vi "Waveform Cluster to Array.vi"(10 "Waveform Cluster":T1) -> (1 "Lengths":i32[](array[numeric]), 2 "Concatenated Waveforms":waveform(dbl)[](array[waveform]))   [LabVIEW 2019, in "Instrument.Lockin.lvlib" / "Instrument.DAQ.lvclass"]
uses:
  Instrument.DAQ.lvclass
  Typedefs/PublicEvents--DAQ.getWaveforms.ctl
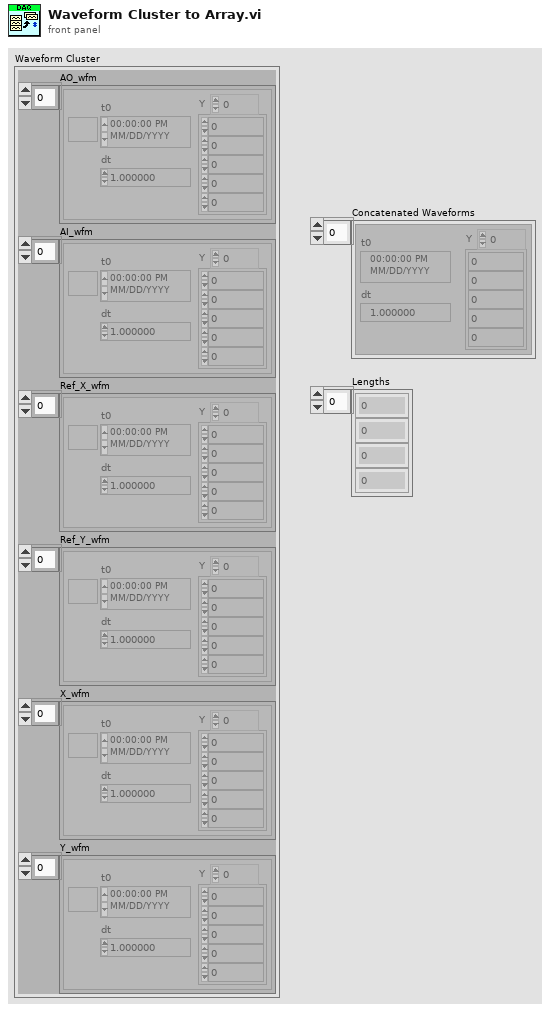
[diagram p1: front panel]
types:
  T1 = typedef "Instrument.Lockin.lvlib/Instrument.DAQ.lvclass/PublicEvents--DAQ.getWaveforms.ctl" = cluster{"AO_wfm":waveform(dbl)[], "AI_wfm":waveform(dbl)[], "Ref_X_wfm":waveform(dbl)[], "Ref_Y_wfm":waveform(dbl)[], "X_wfm":waveform(dbl)[], "Y_wfm":waveform(dbl)[]}
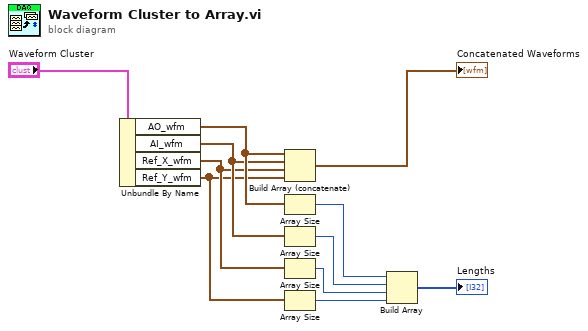
[diagram p0: block diagram]
diagram:
  n1 = Unbundle By Name("Waveform Cluster") -> ("AO_wfm"=w4:waveform(dbl)[], "AI_wfm"=w3:waveform(dbl)[], "Ref_X_wfm"=w2:waveform(dbl)[], "Ref_Y_wfm"=w1:waveform(dbl)[])
  n2 = Build Array (concatenate)(w4, w3, w2, w1) -> (→"Concatenated Waveforms":waveform(dbl)[])
  n3 = Array Size(array=w4) -> (size(s)=w10:i32)
  n4 = Array Size(array=w3) -> (size(s)=w9:i32)
  n5 = Array Size(array=w2) -> (size(s)=w8:i32)
  n6 = Array Size(array=w1) -> (size(s)=w7:i32)
  n7 = Build Array(w10, w9, w8, w7) -> (→"Lengths":i32[])
